vi "import walls.vi"(8 "wall":T1, 9 "empty":T1=1, 11 "Picture path":path) -> (3 "walls/field":T1[][](array[typedef]))   [LabVIEW 2009]
uses:
  square.ctl
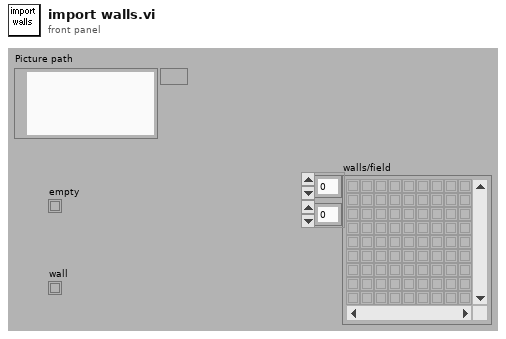
[diagram p1: front panel]
types:
  T1 = typedef "square.ctl" = u8
  T2 = typedef "imagedata.ctl" = cluster{"image type":i32, "image depth":i32, "image":u8[], "mask":u8[], "colors":u32[], "Rectangle":cluster{"left":i16, "top":i16, "right":i16, "bottom":i16}}
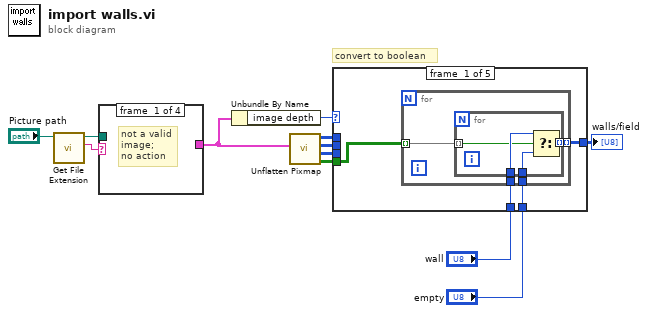
[diagram p0: block diagram]
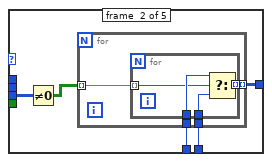
[diagram p2: hidden frame]
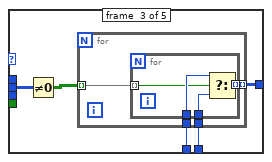
[diagram p3: hidden frame]
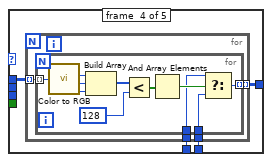
[diagram p4: hidden frame]
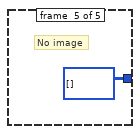
[diagram p5: hidden frame]
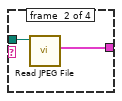
[diagram p6: hidden frame]
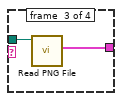
[diagram p7: hidden frame]
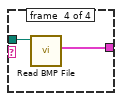
[diagram p8: hidden frame]
diagram:
  # "convert to boolean"
  n1 = call <vilib>:"Get File Extension.vi"("file"="Picture path") -> ("lowercase file extension"=w10:string, "dup file"=w11:path)  [unwired: 7 in, 2 out]
  n2 = case shown="\"png\"" w10 {
    tunnel: w11 -> [_ w14 w16 w18]
    tunnel: [_ w13 w15 w17] -> w9
    frame #0 {
      # "not a valid\nimage;\nno action"
    }
    frame #1 {
      n3 = call <vilib>:"Read JPEG File.vi"("path to JPEG file"=w14) -> ("image data"=w13:T2)  [unwired: 8 in, 2 out]
    }
    frame #2 {
      n4 = call <vilib>:"Read PNG File.vi"("path to PNG file"=w16) -> ("image data"=w15:T2)  [unwired: 8 in, 2 out]
    }
    frame #3 {
      n5 = call <vilib>:"Read BMP File.vi"("path to BMP file"=w18) -> ("image data"=w17:T2)  [unwired: 8 in, 2 out]
    }
  }
  n6 = Unbundle By Name(w9) -> ("image depth"=w8:i32)
  n7 = call <vilib>:"Unflatten Pixmap.vi"("image data"=w9) -> ("1-bit pixmap"=w7:bool[][], "4-bit pixmap"=w4:u8[][], "8-bit pixmap"=w6:u8[][], "24-bit pixmap"=w5:u32[][])  [unwired: 4 in, 3 out]
  n8 = case shown="24, 32" w8 {
    tunnel: w7 -> [w19 _ _ _ _]
    tunnel: w6 -> [_ _ w44 _ _]
    tunnel: w5 -> [_ _ _ w60 _]
    tunnel: w4 -> [_ w32 _ _ _]
    tunnel: "wall" -> [w21 w34 w47 w59 _]
    tunnel: "empty" -> [w22 w35 w48 w58 _]
    tunnel: [w20 w33 w46 w57 T1[][] []] -> w1
    frame #0 {
      n9 = for {
        tunnel: w22 -> [w26]
        tunnel: w21 -> [w25]
        tunnel: [w24] -> w20 mode=indexing
        tunnel: w19 -> [w23] mode=indexing
        n10 = for {
          tunnel: w26 -> [w30]
          tunnel: w25 -> [w29]
          tunnel: [w28] -> w24 mode=indexing
          tunnel: w23 -> [w27] mode=indexing
          n11 = Select(t=w29, s=w27, f=w30) -> (s? t:f=w28:T1)
        }
      }
    }
    frame #1 {
      n12 = Not Equal To 0?(x=w32) -> (x != 0?=w31:bool[][])
      n13 = for {
        tunnel: w35 -> [w39]
        tunnel: w34 -> [w38]
        tunnel: [w37] -> w33 mode=indexing
        tunnel: w31 -> [w36] mode=indexing
        n14 = for {
          tunnel: w39 -> [w43]
          tunnel: w38 -> [w42]
          tunnel: [w41] -> w37 mode=indexing
          tunnel: w36 -> [w40] mode=indexing
          n15 = Select(t=w42, s=w40, f=w43) -> (s? t:f=w41:T1)
        }
      }
    }
    frame #2 {
      n16 = Not Equal To 0?(x=w44) -> (x != 0?=w45:bool[][])
      n17 = for {
        tunnel: w48 -> [w52]
        tunnel: w47 -> [w51]
        tunnel: [w50] -> w46 mode=indexing
        tunnel: w45 -> [w49] mode=indexing
        n18 = for {
          tunnel: w52 -> [w56]
          tunnel: w51 -> [w55]
          tunnel: [w54] -> w50 mode=indexing
          tunnel: w49 -> [w53] mode=indexing
          n19 = Select(t=w55, s=w53, f=w56) -> (s? t:f=w54:T1)
        }
      }
    }
    frame #3 {
      n20 = for {
        tunnel: w60 -> [w64] mode=indexing
        tunnel: w59 -> [w63]
        tunnel: w58 -> [w62]
        tunnel: [w61] -> w57 mode=indexing
        n21 = for {
          tunnel: w64 -> [w75] mode=indexing
          tunnel: w63 -> [w67]
          tunnel: w62 -> [w66]
          tunnel: [w65] -> w61 mode=indexing
          n22 = call <vilib>:"Color to RGB.vi"("Color"=w75) -> ("R"=w74:u8, "G"=w73:u8, "B"=w72:u8)  [unwired: 1 out]
          n23 = Build Array(w74, w73, w72) -> (w71:u8[])
          n24 = Less?(x=w71, y=u8 128) -> (x < y?=w69:bool[])
          n25 = And Array Elements(Boolean array=w69) -> (logical AND=w68:bool)
          n26 = Select(t=w67, s=w68, f=w66) -> (s? t:f=w65:T1)
        }
      }
    }
    frame #4 {
      # "No image"
    }
  }
  "walls/field" <- w1
